vi "Client Writes Complete.vi"(8 "error in":errorcluster, 11 "ClientID in":T1) -> (0 "error out":errorcluster, 3 "ClientID out":T1)   [LabVIEW 2019, in "grpc-lvsupport.lvlib"]
uses:
  grpc-lvsupport.lvlib
  grpcId.ctl
  <vilib>/Utility/file.llb/Application Directory.vi
  <vilib>/Utility/error.llb/Error Cluster From Error Code.vi
  <resource>/labview_grpc_server.dll
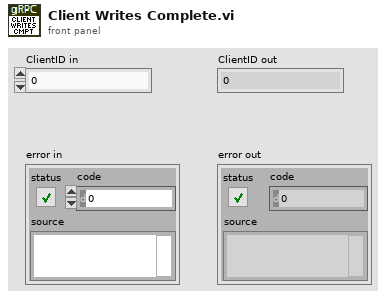
[diagram p1: front panel]
types:
  T1 = typedef "grpc-lvsupport.lvlib/grpcId.ctl" = u64
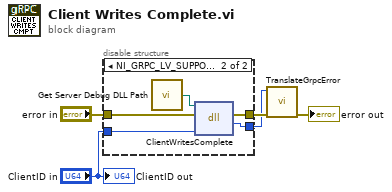
[diagram p0: block diagram]
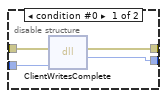
[diagram p2: hidden frame]
diagram:
  n1 = disable-structure shown="NI_GRPC_LV_SUPPORT_DEBUG==True&&RUN_TIME_ENGINE==False" {
    disable-tunnel: "error in" -> [w9 w14]
    disable-tunnel: [w8 w13] -> w4
    disable-tunnel: [w7 w11] -> w2
    disable-tunnel: "ClientID in" -> [w6 w10]
    frame condition #0 {
      n2 = dll-call lib="C:/Program Files (x86)/National Instruments/LabVIEW 2024/resource/labview_grpc_server.*" fn="ClientWritesComplete"(error in=w9, "clientId"=w6) -> (error out=w8:errorcluster, "return type"=w7:i32)  [unwired: 3 in, 1 out]
    }
    frame condition #1 (active) {
      n3 = call "Get Server Debug DLL Path.vi"() -> ("DLL Path"=w12:path)
      n4 = dll-call lib="?" fn="ClientWritesComplete"(path in=w12, error in=w14, "clientId"=w10) -> (error out=w13:errorcluster, "return type"=w11:i32)  [unwired: 2 in, 1 out]
    }
  }
  n5 = call "TranslateGrpcError.vi"("error in"=w4, "Error Code"=w2) -> ("error out"=→"error out":errorcluster)  [unwired: 9 in]
  "ClientID out" <- "ClientID in"
